vi "Rotation Set Modes.vi"   [LabVIEW 2016]
uses:
  Rotation Control Type.ctl
  <vilib>/Rock Robotics/WPI/DriverStation/WPI_DriverStationRobotMode2.ctl
  Rotation Globals.vi
  Robot Global Data.vi
types:
  T1 = typedef "Rotation Control Type.ctl" = enum16{"No Op", "Up", "Down", "Control Up", "Control Down", "Gear Down", "Gear Up"}
  T2 = typedef "WPI_DriverStationRobotMode2.ctl" = enum16{"Autonomous Disabled", "Autonomous Enabled", "Teleop Disabled", "Teleop Enabled", "Disconnected", "Finish", "Test Disabled", "Test Enabled", "Emergency Stopped"}
  T3 = typedef "Rotation Notifier.ctl" = cluster{"Up":bool, "Down":bool, "Rotation Control List":T1, "Control Down":bool, "Manual":bool, "Parameter 1":dbl, "Parameter 2":dbl, "Rotation Notifier":refnum<notifier>, "Step":i32}
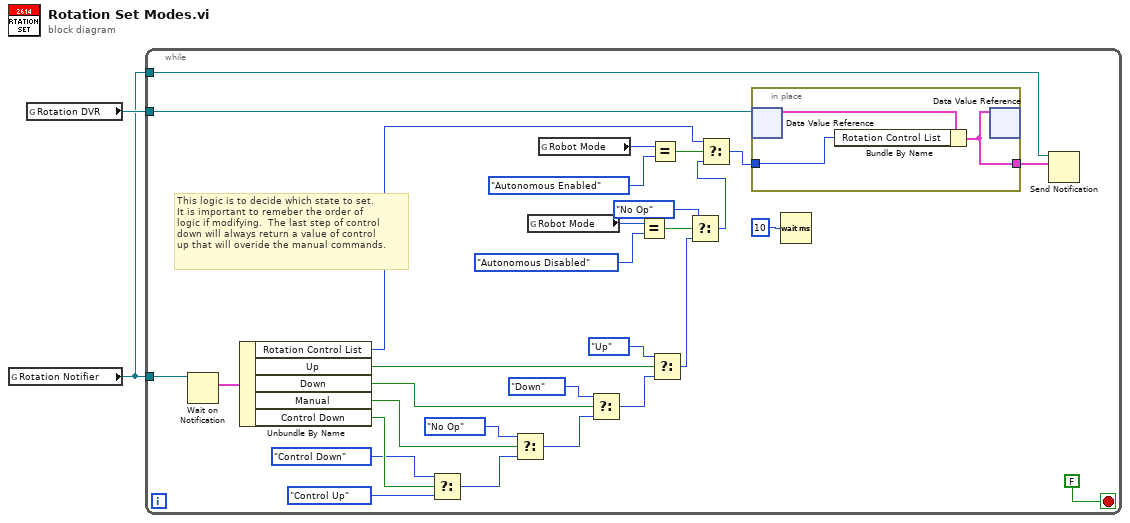
[diagram p0: block diagram]
diagram:
  n1 = global read "Rotation Globals.vi" "Rotation Notifier"() -> (w1:refnum<notifier>)
  n2 = global read "Rotation Globals.vi" "Rotation DVR"() -> (w2:refnum<data-value>)
  n3 = while {
    tunnel: w1 -> [w28]
    tunnel: w2 -> [w27]
    tunnel: w1 -> [w26]
    stop <- FALSE stop-if-true
    # "This logic is to decide which state to set. \nIt is important to remeber the order of \nlogic if modifying.  The last step of control\ndown will always return a value of control \nup that will overide the manual commands."
    n4 = Wait on Notification(notifier=w28) -> (notification=w30:T3)  [unwired: 3 in, 3 out]
    n5 = Unbundle By Name(w30) -> ("Rotation Control List"=w9:T1, "Up"=w29:bool, "Down"=w21:bool, "Manual"=w17:bool, "Control Down"=w20:bool)
    n6 = Select(t=Rotation_Control_Type."Control Down" ("Rotation Control List"), s=w20, f=Rotation_Control_Type."Control Up" ("Rotation Control List")) -> (s? t:f=w16:T1)
    n7 = Select(t=Rotation_Control_Type."No Op", s=w17, f=w16) -> (s? t:f=w15:T1)
    n8 = global read "Robot Global Data.vi" "Robot Mode"() -> (w5:T2)
    n9 = global read "Robot Global Data.vi" "Robot Mode"() -> (w12:T2)
    n10 = Select(t=Rotation_Control_Type."Down" ("Rotation Control List"), s=w21, f=w15) -> (s? t:f=w22:T1)
    n11 = Equal?(x=w5, y=WPI_DriverStationRobotMode2."Autonomous Disabled") -> (x = y?=w4:bool)
    n12 = Equal?(x=w12, y=WPI_DriverStationRobotMode2."Autonomous Enabled") -> (x = y?=w10:bool)
    n13 = Select(t=Rotation_Control_Type."Up" ("Rotation Control List"), s=w29, f=w22) -> (s? t:f=w7:T1)
    n14 = Select(t=Rotation_Control_Type."No Op", s=w4, f=w7) -> (s? t:f=w8:T1)
    n15 = Select(t=w9, s=w10, f=w8) -> (s? t:f=w13:T1)
    n16 = in-place {
      in-place-border: w13 -> [w35]
      in-place-border: [w33] -> w25
      n17 = in-place-dvr #1(w27) -> (w34:T3)  [unwired: 1 out]
      n18 = Bundle By Name(cluster=w34, "Rotation Control List"=w35) -> (w33:T3)
      n19 = in-place-dvr #1(w33) -> ()  [unwired: 2 out]
    }
    n20 = Wait (ms)(milliseconds to wait=u32 10) -> ()  [unwired: 1 out]
    n21 = Send Notification(notification=w25, notifier=w26) -> ()  [unwired: 1 in, 2 out]
  }
